vi "Read Input Registers.vi"(8 "error in":errorcluster, 9 "number of inputs":u16, 10 "starting address":u16, 11 "Master CR in":refnum<class "WebSocket Client CR.lvclass">) -> (0 "error out":errorcluster, 2 "register values":u16[](array[numeric]), 3 "Master CR out":refnum<class "WebSocket Client CR.lvclass">)   [LabVIEW 2021]
doc: "Reads <B>number of inputs</B> input registers starting at <B>starting address</B> from the device."
uses:
  WebSocket Client CR.lvclass
  WebSocket Client CR.lvclass/WebSocket Client CR.ctl
  Modbus_v121c/Data Model/Device Data Model.lvclass
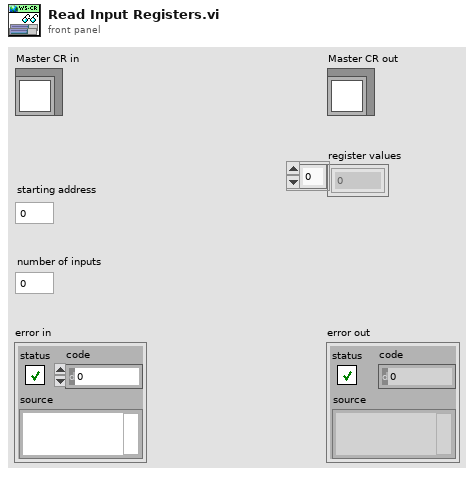
[diagram p1: front panel]
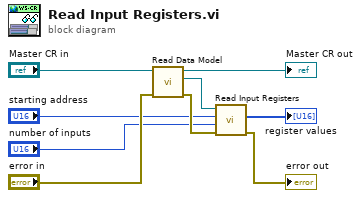
[diagram p0: block diagram]
diagram:
  n1 = call "Read Data Model.vi"("error in (no error)"="error in", "Master CR in"="Master CR in") -> ("error out"=w6:errorcluster, "Data Model"=w7:refnum<class "Device Data Model.lvclass">, "Master CR out"=→"Master CR out":refnum<class "WebSocket Client CR.lvclass">)  [unwired: 7 in]
  n2 = call-dynamic "Read Input Registers.vi"("error in"=w6, "number of registers"="number of inputs", "starting address"="starting address", "device data model in"=w7) -> ("error out"=→"error out":errorcluster, "data"=→"register values":u16[])  [unwired: 5 in, 1 out]
